vi "__SIS_Mag_Get.vi"(10 "Bias_LO_equip":T1={"Node address"=19, "CAN Interface"="CAN0", "Cartridge band"=10, "Slave Node in"={"Address"=0, "Serial Number"=[]}, "ObjHandle out"=0, "POL"=1, "sb"=1, "GPIB_SM (SIS S,V)"="24", "GPIB_DMM (SIS I)"="22", "GPIB_SM (MAG I) "="25", "GPIB_SG(LO)"="19", "GPIB_PW (PAMP) "="6", "GPIB_TMP1(8ch)"="12", "GPIB_TMP2(2ch)  "="13", "WCA_avg"=10, "Rsen"=10.0, "BiasModule"=1, "LOModule "=1, "WCA_LO_FREQ_SET"={"YTO Low freq. [GHz]"=14.42, "YTO High freq. [GHz]"=17.7, "Kvco"=1, "Lock Pol."=0, "SET LO FREQ"=72.5, "Multiplier"=6.0, "YTO (HEX)"=0, "YTO coarse( FREQ)"=25.0, "NULL PLL INTEGRATOR"=FALSE}, "Res for"=0} {"Res for" items=["none", "series res", "parallel res"]; "WCA_LO_FREQ_SET"."YTO coarse( FREQ)" min=25 max=150 step=0.0001 format="%.3f"; "WCA_LO_FREQ_SET"."Multiplier" min=3 max=6 step=3; "WCA_LO_FREQ_SET"."SET LO FREQ" min=25 max=150 step=0.0001 format="%.3f"; "WCA_LO_FREQ_SET"."Lock Pol." items=["Lower", "Upper"]; "WCA_LO_FREQ_SET"."Kvco" items=["7.5MHz/V", "15MHz/V"]; "WCA_LO_FREQ_SET"."YTO High freq. [GHz]" format="%.3f"; "WCA_LO_FREQ_SET"."YTO Low freq. [GHz]" format="%.3f"; "LOModule" items=["Manual", "B10Lab LO", "WCA LO"]; "BiasModule" items=["B10Lab Bias", "WCA BiasModule"]; "Slave Node in"."Serial Number" format="%.0x"; "Slave Node in"."Address" format="%.0x"; "Cartridge band" max=10 step=1; "Node address" format="%.0x"}) -> (1 "Get_Mag_I":dbl, 3 "Get_Mag_V":dbl)   [LabVIEW 2017]
panel:
  # "LO freq. [GHz]"
  # "YTO LOW\n/High Freq."
  # "ZERO Intgrtr"
  # "Node Address"
  # "Serial Number"
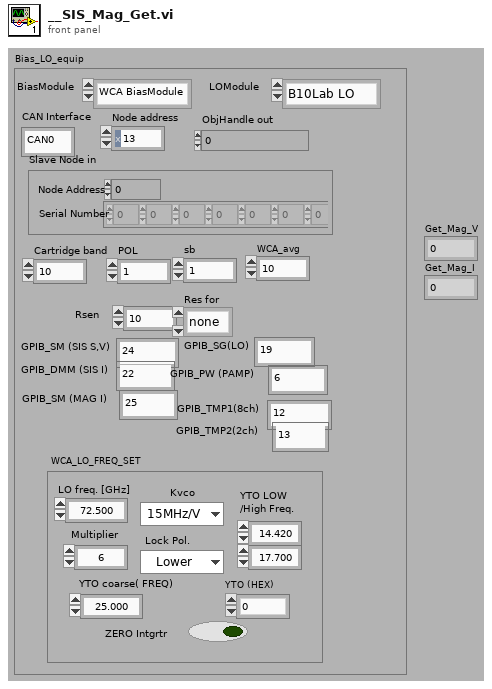
[diagram p1: front panel]
types:
  T1 = cluster{"Node address":u16, "CAN Interface":string, "Cartridge band":u32, "Slave Node in":cluster{"Address":i16, "Serial Number":i8[]}, "ObjHandle out":u32, "POL":u32, "sb":u32, "GPIB_SM (SIS S,V)":string, "GPIB_DMM (SIS I)":string, "GPIB_SM (MAG I) ":string, "GPIB_SG(LO)":string, "GPIB_PW (PAMP) ":string, "GPIB_TMP1(8ch)":string, "GPIB_TMP2(2ch)  ":string, "WCA_avg":i32, "Rsen":dbl, "BiasModule":u16, "LOModule ":u16, "WCA_LO_FREQ_SET":cluster{"YTO Low freq. [GHz]":sgl, "YTO High freq. [GHz]":sgl, "Kvco":u16, "Lock Pol.":u16, "SET LO FREQ":sgl, "Multiplier":sgl, "YTO (HEX)":u16, "YTO coarse( FREQ)":sgl, "NULL PLL INTEGRATOR":bool}, "Res for":u16}
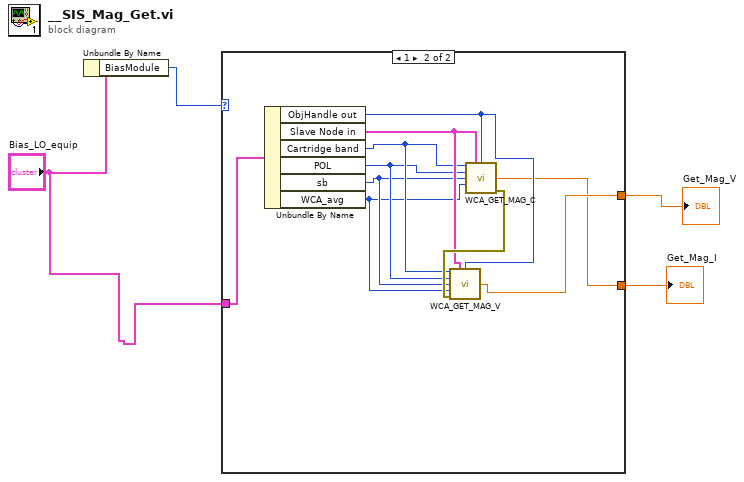
[diagram p0: block diagram]
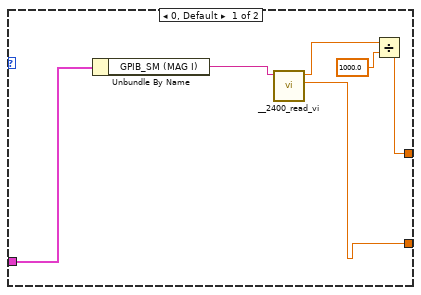
[diagram p2: hidden frame]
diagram:
  n1 = Unbundle By Name("Bias_LO_equip") -> ("BiasModule"=w1:u16)
  n2 = case shown="1" w1 {
    tunnel: "Bias_LO_equip" -> [w10 w20]
    tunnel: [w5 w12] -> w4
    tunnel: [w8 w11] -> w3
    frame 0, Default {
      n3 = Unbundle By Name(w10) -> ("GPIB_SM (MAG I)"=w9:string)
      n4 = call "__2400_read_vi.vi"("GPIB"=w9) -> ("volt_current (mA)"=w8:dbl, "volt_read (mV)"=w7:dbl)  [unwired: 4 in, 1 out]
      n5 = Divide(x=w7, y=1000.0) -> (x/y=w5:dbl)
    }
    frame 1 {
      n6 = Unbundle By Name(w20) -> ("ObjHandle out"=w18:u32, "Slave Node in"=w17:cluster{"Address":i16, "Serial Number":i8[]}, "Cartridge band"=w16:u32, "POL"=w15:u32, "sb"=w14:u32, "WCA_avg"=w13:i32)
      n7 = call "WCA_GET_MAG_C.vi"("Cartridge Band"=w16, "Slave Node in"=w17, "ObjHandle in"=w18, "POL"=w15, "sb"=w14, "avg"=w13) -> ("GET_MAG_C"=w11:dbl, "error out"=w19:errorcluster)  [unwired: 7 in, 1 out]
      n8 = call "WCA_GET_MAG_V.vi"("Cartridge Band"=w16, "Slave Node in"=w17, "ObjHandle in"=w18, "POL"=w15, "sb"=w14, "avg"=w13, "error in (no error)"=w19) -> ("GET_MAG_V"=w12:dbl)  [unwired: 6 in, 2 out]
    }
  }
  "Get_Mag_V" <- w4
  "Get_Mag_I" <- w3
